vi "Write Bob Enq.vi"(8 "error in (no error)":errorcluster, 10 "Actor Framework:Message Enqueuer":refnum<class "Message Enqueuer.lvclass">, 11 "Alice in":refnum<class "Alice.lvclass">) -> (0 "error out":errorcluster, 3 "Alice out":refnum<class "Alice.lvclass">)   [LabVIEW 2014, in "Alice.lvlib" / "Alice.lvclass"]
uses:
  Alice.lvclass
  <vilib>/ActorFramework/Message Enqueuer/Message Enqueuer.lvclass
  Alice.lvclass/Alice.ctl
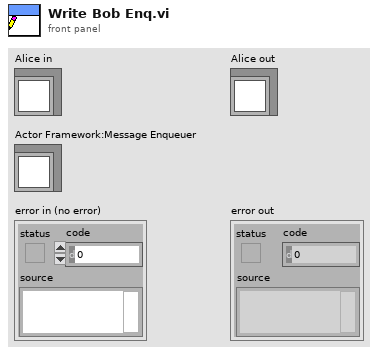
[diagram p1: front panel]
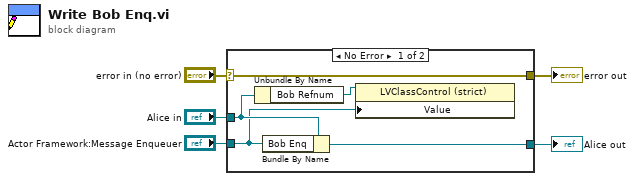
[diagram p0: block diagram]
diagram:
  n1 = case shown="No Error" "error in (no error)" {
    selector: "error in (no error)" -> [w10 w11]
    tunnel: [w10 w11] -> w4
    tunnel: [w9 w12] -> w2
    tunnel: "Alice in" -> [w8 w12]
    tunnel: "Actor Framework:Message Enqueuer" -> [w6 _]
    frame No Error {
      n2 = Unbundle By Name(w8) -> ("Bob Refnum"=w7:refnum<vi>)
      n3 = Bundle By Name(cluster=w8, "Bob Enq"=w6) -> (w9:refnum<class "Alice.lvclass">)
      n4 = property class="LVClassControl (strict)"(reference=w7, "Value"=w6) -> ()  [unwired: 1 in, 2 out]
    }
    frame Error {
    }
  }
  "error out" <- w4
  "Alice out" <- w2
